vi "Add Point.vi"(8 "error in (no error)":errorcluster, 9 "Y":dbl, 10 "X":dbl, 11 "Data2D in":refnum<class "Data2D.lvclass">) -> (0 "error out":errorcluster, 3 "Data2D out":refnum<class "Data2D.lvclass">)   [LabVIEW 2018, in "Data2D.lvclass"]
uses:
  Data2D.lvclass
  Data2D.lvclass/Data2D.ctl
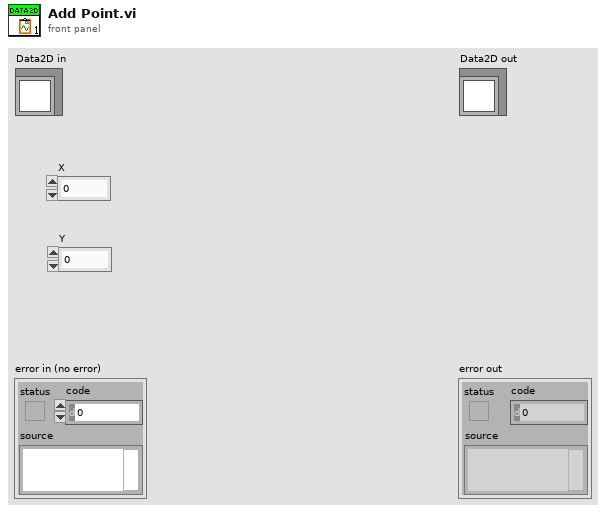
[diagram p1: front panel]
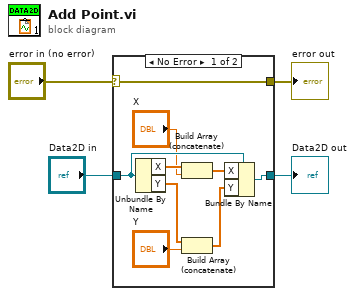
[diagram p0: block diagram]
diagram:
  n1 = case shown="No Error" "error in (no error)" {
    selector: "error in (no error)" -> [w13 w15]
    tunnel: [w13 w15] -> w3
    tunnel: [w12 w14] -> w1
    tunnel: "Data2D in" -> [w11 w14]
    frame No Error {
      n2 = Unbundle By Name(w11) -> ("X"=w10:dbl[], "Y"=w7:dbl[])
      n3 = Build Array (concatenate)(w10, "X") -> (w8:dbl[])
      n4 = Build Array (concatenate)(w7, "Y") -> (w5:dbl[])
      n5 = Bundle By Name(cluster=w11, "X"=w8, "Y"=w5) -> (w12:refnum<class "Data2D.lvclass">)
    }
    frame Error {
    }
  }
  "error out" <- w3
  "Data2D out" <- w1
